vi "hmac_str.vi"(0 "Method":string, 5 "Nonce":string, 7 "Date":string, 9 "ctype":string, 11 "path":string) -> (4 "hmac_str":string, 8 "hmac_str":u8[](array[numeric]))   [LabVIEW 2019]
panel:
  out "length":i32
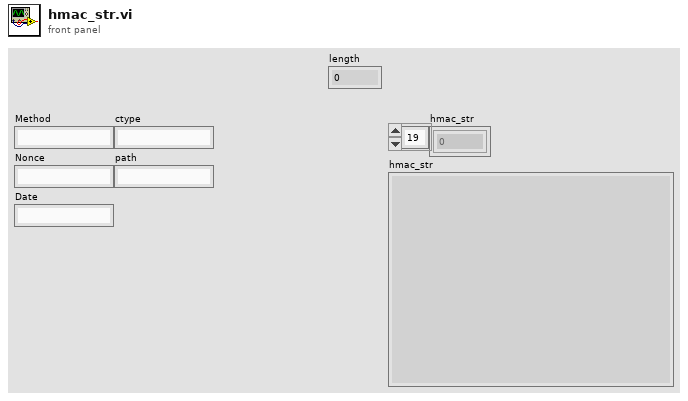
[diagram p1: front panel]
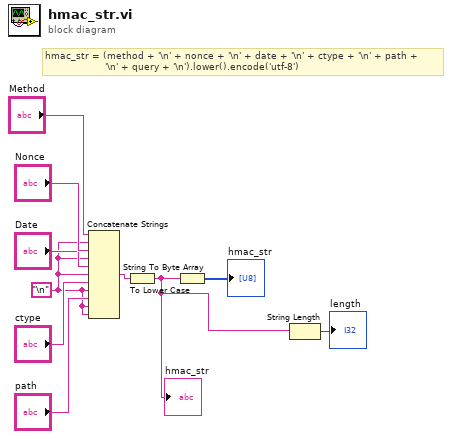
[diagram p0: block diagram]
diagram:
  w1 = "\n"
  # "hmac_str = (method + '\\n' + nonce + '\\n' + date + '\\n' + ctype + '\\n' + path +\n                    '\\n' + query + '\\n').lower().encode('utf-8')"
  n1 = Concatenate Strings("Method", w1, "Nonce", w1, "Date", w1, "ctype", w1, "path", w1, w1) -> (w5:string)
  n2 = To Lower Case(string=w5) -> (all lower case string=w3:string)
  "hmac_str" <- w3
  n3 = String To Byte Array(string=w3) -> (unsigned byte array=→"hmac_str":u8[])
  n4 = String Length(string=w3) -> (length=→"length":i32)
